vi "DetectDrift (SubVI).vi"(0 "Application in":refnum<vi>, 7 "Drift Correction image":dbl[][][](array[numeric]), 12 "Settings in":T1={"Drift Correction Settings"={"Drift Correction every"=80, "Drift correction Pixels"=256, "Channel index (0-23)"=0, "MaxImagesBack"=2, "Threshold"=2, "Increment"=8, "max applied Drift Correction"=20, "Correct Drift"=TRUE, "Correlate"=0, "Correct z drift"=FALSE, "zdrift \nDuration (s)"=0.0}, "Spectroscopy Setting"={"Imaging Current"=1e-11, "ref Current"=7e-11, "tip Speed (m/s)"=2e-09, "Imaging Bias"=0.02, "ref Bias"=-0.1, "preSTS delay [ms]"=500, "STS z offset"=2e-10, "during Spec Bias (V)"=-0.1, "trigger1 < Hz"=0.0, "trigger 2 >Hz"=0.0, "autoStop"=FALSE, "Spectroscopy"=0, "PLL ON/OFF"=TRUE, "readjust setpoint every "=1, "z Reference"=FALSE, "Lock In"=TRUE}, "Misc"={"File name"="symmetric_node_zOff=200p", "Email when finished"="cornelius.krull@monash.edu,Dhaneesh.Gopalakrishnan@monash.edu,marina.castelli@monash.edu"}, "Grid Settings"={"type"=1, "type order"=1, "X pixel"=0, "Y pixel"=0, "Grid_Parms"={"center X (m)"=0.0, "center Y (m)"=0.0, "width (m)"=0.0, "height (m)"=0.0, "angle (deg)"=0.0}}} {"Grid Settings"."type order" items=["Line", "Grid"]; "Grid Settings"."type" items=["Line", "Grid"]; "Spectroscopy Setting"."Spectroscopy" items=["Bias", "zSpec"]; "Spectroscopy Setting"."trigger 2 >Hz" format="%#_6p"; "Spectroscopy Setting"."trigger1 < Hz" format="%#_6p"; "Spectroscopy Setting"."during Spec Bias (V)" format="%#_5p"; "Spectroscopy Setting"."STS z offset" format="%#_6p"; "Spectroscopy Setting"."ref Bias" format="%#_6p"; "Spectroscopy Setting"."Imaging Bias" format="%#_6p"; "Spectroscopy Setting"."tip Speed (m/s)" format="%.2p"; "Spectroscopy Setting"."ref Current" format="%#_6p"; "Spectroscopy Setting"."Imaging Current" format="%#_6p"; "Drift Correction Settings"."Correlate" items=["first Frame", "successive Frames"]; "Drift Correction Settings"."max applied Drift Correction" min=1 max=100 step=1 format="%.0p"; "Drift Correction Settings"."Threshold" min=1 step=1; "Drift Correction Settings"."Channel index (0-23)" items=["Current"=0, "Z (m)"=14]}) -> (1 "x drift":sgl, 2 "y drift":sgl, 3 "z drift":dbl, 4 "Application out":refnum<vi>, 10 "XY Drift?":bool)   [LabVIEW 2021]
uses:
  <userlib>/Nanonis Prog Interface V5/Nanonis Prog Interface.lvlib
panel:
  # "z Spectroscopy"
  # "GRID points"
  # "Increase this if no Drift was detected for \na certain number of images"
  # "% of image size"
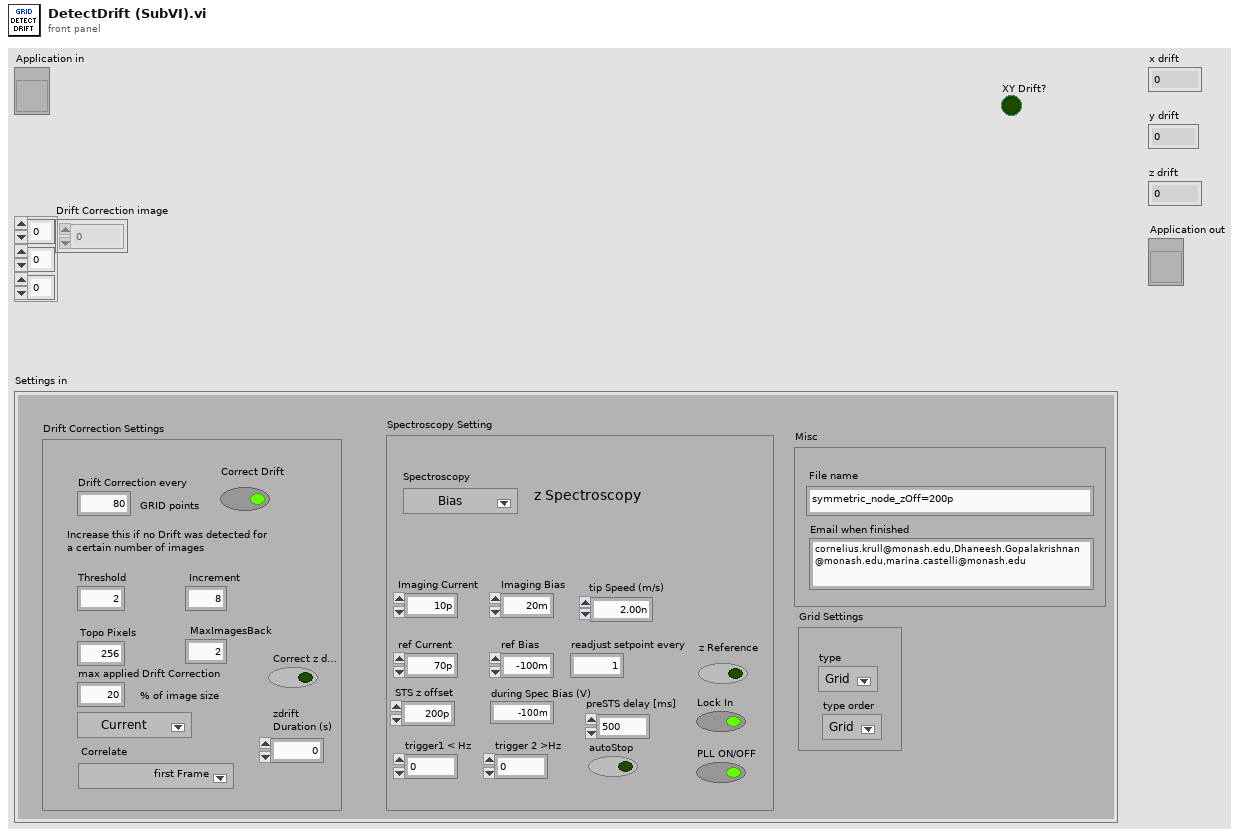
[diagram p1: front panel]
types:
  T1 = cluster{"Drift Correction Settings":cluster{"Drift Correction every":i32, "Drift correction Pixels":i32, "Channel index (0-23)":u8, "MaxImagesBack":i32, "Threshold":i32, "Increment":i32, "max applied Drift Correction":i32, "Correct Drift":bool, "Correlate":u16, "Correct z drift":bool, "zdrift \nDuration (s)":dbl}, "Spectroscopy Setting":cluster{"Imaging Current":dbl, "ref Current":dbl, "tip Speed (m/s)":sgl, "Imaging Bias":dbl, "ref Bias":dbl, "preSTS delay [ms]":u32, "STS z offset":dbl, "during Spec Bias (V)":sgl, "trigger1 < Hz":sgl, "trigger 2 >Hz":sgl, "autoStop":bool, "Spectroscopy":u16, "PLL ON/OFF":bool, "readjust setpoint every ":i32, "z Reference":bool, "Lock In":bool}, "Misc":cluster{"File name":string, "Email when finished":string}, "Grid Settings":cluster{"type":u16, "type order":u16, "X pixel":i32, "Y pixel":i32, "Grid_Parms":cluster{"center X (m)":sgl, "center Y (m)":sgl, "width (m)":sgl, "height (m)":sgl, "angle (deg)":sgl}}}
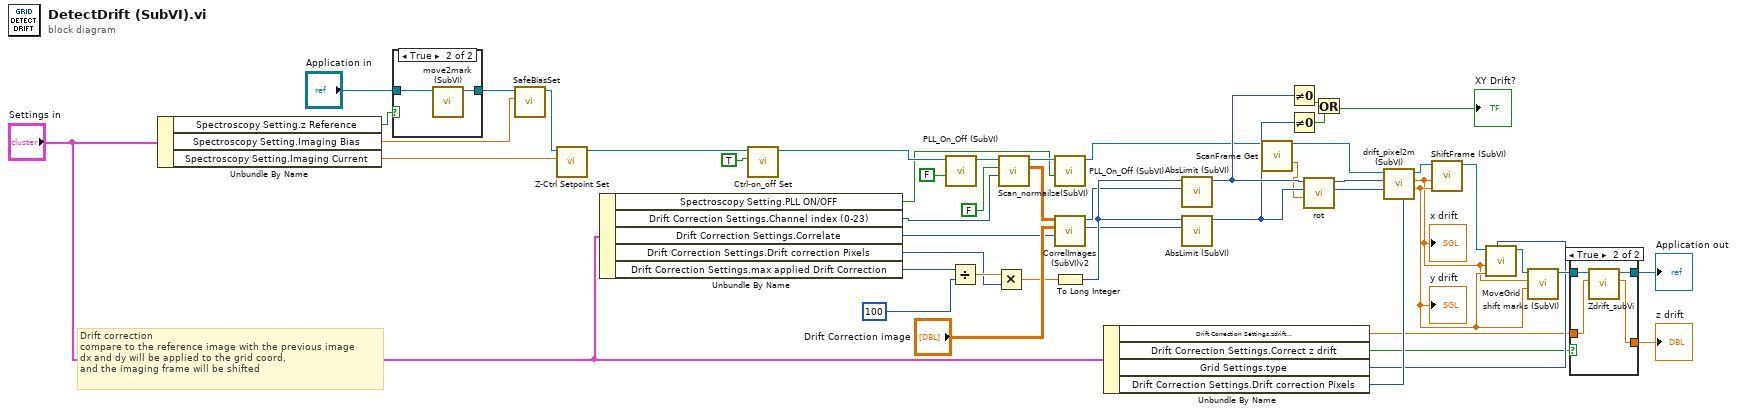
[diagram p0: block diagram]
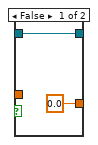
[diagram p3: hidden frame]
diagram:
  # "Drift correction \ncompare to the reference image with the previous image \ndx and dy will be applied to the grid coord, \nand the imaging frame will be shifted"
  n1 = Unbundle By Name("Settings in") -> ("Spectroscopy Setting.z Reference"=w47:bool, "Spectroscopy Setting.Imaging Bias"=w45:dbl, "Spectroscopy Setting.Imaging Current"=w46:dbl)
  n2 = case shown="True" w47 {
    tunnel: "Application in" -> [w50 w52]
    tunnel: [w50 w51] -> w38
    frame False {
    }
    frame True {
      n3 = call "move2mark (SubVI).vi"("Application in"=w52) -> ("Application out"=w51:refnum<vi>)  [unwired: 10 in]
    }
  }
  n4 = call "SafeBiasSet.vi"("Application ref in"=w38, "Bias (V)"=w45) -> ("Application ref out"=w32:refnum<vi>)  [unwired: 7 in, 1 out]
  n5 = call <userlib>:"Z-Ctrl Setpoint Set.vi"("Z Controller setpoint"=w46, "Application ref in"=w32) -> ("Application ref out"=w39:refnum<vi>)  [unwired: 8 in, 1 out]
  n6 = Unbundle By Name("Settings in") -> ("Spectroscopy Setting.PLL ON/OFF"=w11:bool, "Drift Correction Settings.Channel index (0-23)"=w18:u8, "Drift Correction Settings.Correlate"=w19:u16, "Drift Correction Settings.Drift correction Pixels"=w16:i32, "Drift Correction Settings.max applied Drift Correction"=w49:i32)
  n7 = call <userlib>:"Ctrl-on_off Set.vi"("Z Controller ON/OFF"=TRUE, "Application ref in"=w39) -> ("Application ref out"=w41:refnum<vi>)  [unwired: 8 in, 1 out]
  n8 = call "PLL_On_Off (SubVI).vi"("Output ON/OFF (F=OFF)"=FALSE, "Application in"=w41) -> ("Application out"=w42:refnum<vi>)  [unwired: 8 in, 1 out]
  n9 = Divide(x=w49, y=100) -> (x/y=w27:dbl)
  n10 = Multiply(x=w27, y=w16) -> (x*y=w26:dbl)
  n11 = call "Scan_normailze(SubVI).vi"("Channel index (0-23)"=w18, "Normalization"=FALSE ("Boolean"), "Application in"=w42) -> ("Array"=w23:dbl[][], "Application out"=w44:refnum<vi>)  [unwired: 6 in, 1 out]
  n12 = call "PLL_On_Off (SubVI).vi"("Output ON/OFF (F=OFF)"=w11, "Application in"=w44) -> ("Application out"=w3:refnum<vi>)  [unwired: 8 in, 1 out]
  n13 = call "CorrelImages (SubVI)v2.vi"("Correlate"=w19, "Ref Array"="Drift Correction image", "New Image"=w23) -> ("Y drift"=w29:i32, "X drift"=w30:i32)  [unwired: 5 in, 2 out]
  n14 = To Long Integer(number=w26) -> (32bit integer=w31:i32)
  n15 = Unbundle By Name("Settings in") -> ("Drift Correction Settings.zdrift \nDuration (s)"=w12:dbl, "Drift Correction Settings.Correct z drift"=w13:bool, "Grid Settings.type"=w14:u16, "Drift Correction Settings.Drift correction Pixels"=w15:i32)
  n16 = call "AbsLimit (SubVI).vi"("in"=w30, "Abslimt"=w31) -> ("Numeric out"=w7:i32)  [unwired: 9 in]
  n17 = call "AbsLimit (SubVI).vi"("in"=w29, "Abslimt"=w31) -> ("Numeric out"=w5:i32)  [unwired: 9 in]
  n18 = call <userlib>:"ScanFrame Get.vi"("Application ref in"=w3) -> ("Application ref out"=w2:refnum<vi>, "Angle (deg)"=w1:sgl)  [unwired: 10 in, 3 out]
  n19 = Not Equal To 0?(x=w7) -> (x != 0?=w10:bool)
  n20 = Not Equal To 0?(x=w5) -> (x != 0?=w9:bool)
  n21 = call "rot.vi"("angle"=w1, "y"=w5, "x"=w7) -> ("y'"=w4:i32, "x'"=w6:i32)  [unwired: 7 in]
  n22 = Or(x=w10, y=w9) -> (x .or. y?=→"XY Drift?":bool)
  n23 = call "drift_pixel2m (SubVI).vi"("Application in"=w2, "X drift"=w6, "Y drift"=w4, "Drift correction Pixels"=w15) -> ("Application out"=w25:refnum<vi>, "x drift"=w34:sgl, "y drift"=w35:sgl)  [unwired: 2 in, 1 out]
  "y drift" <- w35
  "x drift" <- w34
  n24 = call "ShiftFrame (SubVI).vi"("Y shift"=w35, "X shift"=w34, "Application in"=w25) -> ("Application out"=w24:refnum<vi>)  [unwired: 8 in]
  n25 = call "MoveGrid.vi"("type"=w14, "y"=w35, "x"=w34, "Application ref in"=w24) -> ("Application ref out"=w36:refnum<vi>)  [unwired: 6 in, 1 out]
  n26 = call "shift marks (SubVI).vi"("y"=w35, "x"=w34, "Application in"=w36) -> ("Application out"=w37:refnum<vi>)  [unwired: 7 in, 1 out]
  n27 = case shown="True" w13 {
    tunnel: [0.0 ("z drift") w58] -> w21
    tunnel: w37 -> [w53 w57]
    tunnel: [w53 w56] -> w22
    tunnel: w12 -> [_ w55]
    frame False {
    }
    frame True {
      n28 = call "Zdrift_subVi.vi"("Duration"=w55, "Application in"=w57) -> ("z drift"=w58:dbl, "Application out"=w56:refnum<vi>)  [unwired: 7 in, 1 out]
    }
  }
  "Application out" <- w22
  "z drift" <- w21
